vi "Image Caption.vi"(0 "PDF Report IN":T21(xcontrol), 9 "Caption IN":string, 11 "error IN":errorcluster) -> (4 "PDF Report OUT":T21(xcontrol), 6 "Paragraph Refnum":refnum<k24>, 15 "error OUT":errorcluster)   [LabVIEW 2013]
doc: "Version 1.0\nDeveloped by Jean-Marc Simard\nCopyright © 2010, Exaprom Inc.\nAll rights reserved.\nLicense: BSD\n\nWith iTextSharp 4.1.6 (http://itextsharp.sourceforge.net)\nunder Mozilla Public License Version 1.1\n(http://www.mozilla.org/MPL/MPL-1.1.html)"
uses:
  Controls/PDF Report Xcontrol/PDF Report.xctl
  C:/Users/MaxCorp/Documents/GitHub/TopView/DLL/itextsharp.dll
  DLL/itextsharp.dll
  Controls/Paragraphe cluster.ctl
  Controls/Texte alignement.ctl
  Controls/Line spacing.ctl
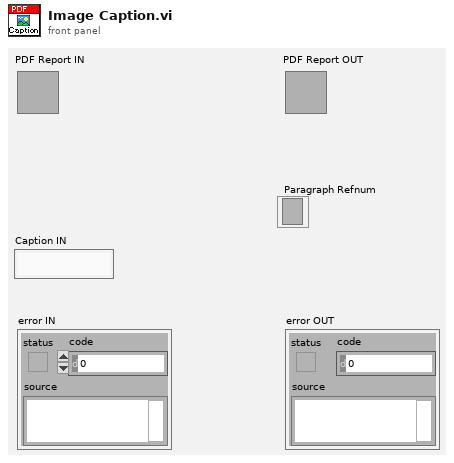
[diagram p1: front panel]
types:
  T1 = typedef "Font cluster.ctl" = cluster{"Name":string, "Size":T2, "Color":T3, "Style":cluster{"Bold":bool, "Italic":bool, "Underline":bool, "Strikeout":bool}}
  T2 = typedef "Font size.ctl" = sgl
  T3 = typedef "Font color.ctl" = u32
  T4 = typedef "Unit.ctl" = enum16{"inch", "mm"}
  T5 = typedef "Paragraphe cluster.ctl" = cluster{" Aligment":T6, "Line spacing":T7}
  T6 = typedef "Texte alignement.ctl" = enum16{"Select", "CENTER", "JUSTIFY", "LEFT", "RIGHT"}
  T7 = typedef "Line spacing.ctl" = enum16{"Select", "1.0", "1.5", "2.0"}
  T8 = typedef "Page dimensions.ctl" = cluster{"Start at page":i32, "Orientation":T9, "widht":sgl, "height":sgl, "Margin left":sgl, "Margin right":sgl, "Margin top":sgl, "Margin bottom":sgl}
  T9 = typedef "Page Orientation.ctl" = enum16{"Portrait", "Landscape"}
  T10 = typedef "Image or Table Caption.ctl" = cluster{"Caption":string, "Separator":string, "Position":enum16{"Above", "Below"}}
  T11 = typedef "Header Footer [ ].ctl" = T12[]
  T12 = typedef "Header Footer cluster.ctl" = cluster{"Start page":i32, "Type":T13, "Alignment":T14, "Vertical Alignement":T15, "Image (%)":sgl, "Page #":T16, "Text":string, "Path":string, "Font":T1, "Font refnum":refnum<k24>, "Line":cluster{"Line":T17, "Thickness (points)":sgl, "Colour":T3}}
  T13 = typedef "Header Footer Type.ctl" = enum16{"Select", "Text", "Text + hyperlink", "Page number", "Image", "Image + hyperlink"}
  T14 = typedef "Header footer horiz alignment.ctl" = enum16{"Left", "Center", "Right"}
  T15 = typedef "Cell Vertical alignment.ctl" = enum16{"TOP", "MIDDLE", "BOTTOM"}
  T16 = typedef "Page number.ctl" = cluster{"Text 1":string, "Text 2":string, "Text 3":string}
  T17 = typedef "Header Footer Line.ctl" = enum16{"No line", "Horizontal line"}
  T18 = typedef "Watermark cluster2.ctl" = cluster{"Show? (F)":bool, "Type":enum16{"Image", "Text"}, "Opacity (%)":sgl, "Rotate(°)":sgl, "Position":cluster{"Position":T19, "X":sgl, "Y":sgl}, "Image path":path, "Scaled(%)":sgl, "Image refnum":refnum<k24>, "Text":string, "Font":cluster{"Name":string, "Size":T2, "Color":T3}, "Font refnum":refnum<k24>, "Alignment":T14, "Automatic":bool}
  T19 = typedef "Watermark Position.ctl" = enum16{"Absolute", "Center (page)", "Center (text section)"}
  T20 = typedef "System Fonts.ctl" = cluster{"Font name [ ]":string[], "Font and file names [ ]":cluster{"Font name":string, "File name":string}[]}
  T21 = cluster{"Document":refnum<k24>, "Writer":refnum<k24>, "Default Font":refnum<k24>, "Default Font cluster":T1, "Path":path, "Unit (default = mm)":T4, "Paragraphe cluster":T5, "Pages dimensions [ ]":T8[], "Captions":cluster{"Image":T10, "Image counter":u16, "Table":T10, "Table counter":u16, "Font":T1}, "Header":T11, "Footer":T11, "Watermark ":T18, "Actual VI name":string, "System Fonts":T20}
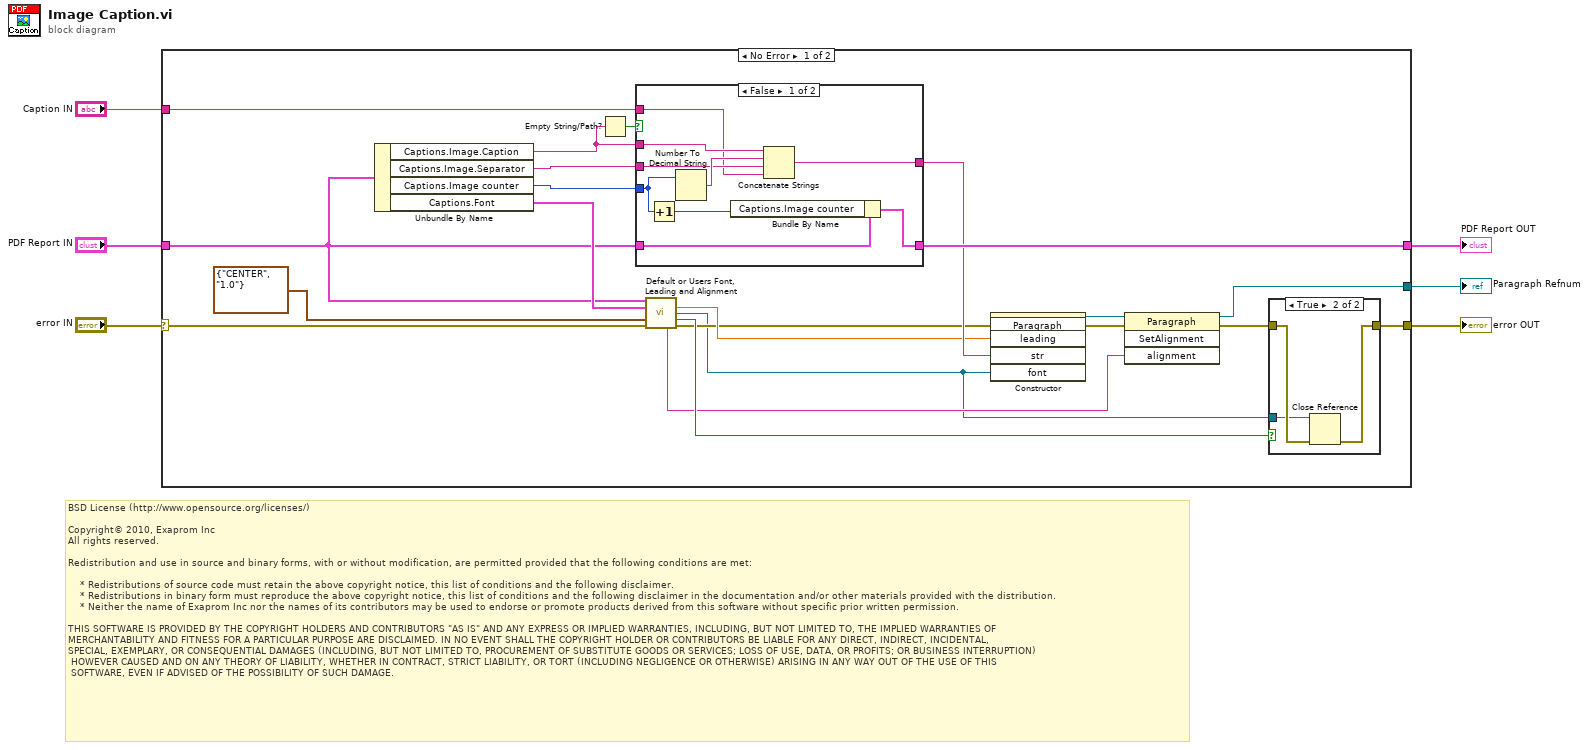
[diagram p0: block diagram]
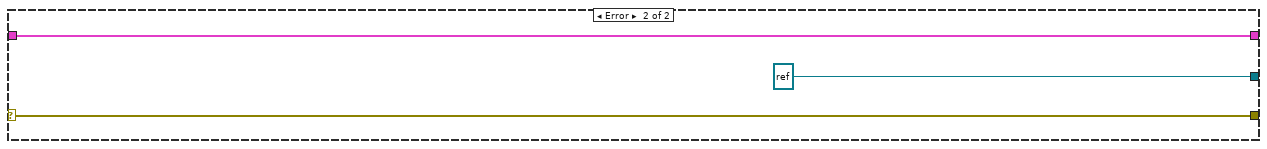
[diagram p4: hidden frame]
diagram:
  # "BSD License (http://www.opensource.org/licenses/)\n\nCopyright© 2010, Exaprom Inc\nAll rights reserved.\n\nRedistribution and use in source and binary forms, with or without modification, are permitted provided that the following conditions are met:\n\n    * Redistributions of source code must retain the above copyright notice, this list of conditions and the following disclaimer.\n    * Redistributions in binary form must reproduce the above copyright notice, this list of conditions and the following disclaimer in the documentation and/or other materials provided with the distribution.\n    * Neither the name of Exaprom Inc nor the names of its contributors may be used to endorse or promote products derived from this software without specific prior written permission.\n\nTHIS SOFTWARE IS PROVIDED BY THE COPYRIGHT HOLDERS AND CONTRIBUTORS \"AS IS\" AND ANY EXPRESS OR IMPLIED WARRANTIES, INCLUDING, BUT NOT LIMITED TO, THE IMPLIED WARRANTIES OF \nMERCHANTABILITY AND FITNESS FOR A PARTICULAR PURPOSE ARE DISCLAIMED. IN NO EVENT SHALL THE COPYRIGHT HOLDER OR CONTRIBUTORS BE LIABLE FOR ANY DIRECT, INDIRECT, INCIDENTAL,\nSPECIAL, EXEMPLARY, OR CONSEQUENTIAL DAMAGES (INCLUDING, BUT NOT LIMITED TO, PROCUREMENT OF SUBSTITUTE GOODS OR SERVICES; LOSS OF USE, DATA, OR PROFITS; OR BUSINESS INTERRUPTION)\n HOWEVER CAUSED AND ON ANY THEORY OF LIABILITY, WHETHER IN CONTRACT, STRICT LIABILITY, OR TORT (INCLUDING NEGLIGENCE OR OTHERWISE) ARISING IN ANY WAY OUT OF THE USE OF THIS\n SOFTWARE, EVEN IF ADVISED OF THE POSSIBILITY OF SUCH DAMAGE."
  n1 = case shown="No Error" "error IN" {
    selector: "error IN" -> [w17 w45]
    tunnel: [w26 w44] -> w6
    tunnel: "Caption IN" -> [w22 _]
    tunnel: "PDF Report IN" -> [w16 w44]
    tunnel: [w19 w45] -> w3
    tunnel: [w7 refnum<k24> refnum ("new reference")] -> w1
    frame No Error {
      n2 = Unbundle By Name(w16) -> ("Captions.Image.Caption"=w23:string, "Captions.Image.Separator"=w24:string, "Captions.Image counter"=w25:u16, "Captions.Font"=w27:T1)
      n3 = Empty String/Path?(string/path=w23) -> (empty?=w21:bool)
      n4 = case shown="False" w21 {
        tunnel: w22 -> [w37 w42]
        tunnel: w23 -> [w40 _]
        tunnel: w24 -> [w38 _]
        tunnel: w25 -> [w36 _]
        tunnel: [w32 w42] -> w13
        tunnel: w16 -> [w35 w41]
        tunnel: [w33 w41] -> w26
        frame False {
          n5 = Increment(x=w36) -> (x+1=w34:u16)
          n6 = Number To Decimal String(number=w36) -> (decimal integer string=w39:string)  [unwired: 1 out]
          n7 = Bundle By Name(cluster=w35, "Captions.Image counter"=w34) -> (w33:T21)
          n8 = Concatenate Strings(w40, w39, w38, w37) -> (w32:string)
        }
        frame True {
        }
      }
      n9 = call "Default or Users Font, Leading and Alignment.vi"("PDF Report"=w16, "Font"=w27, "Paragraphe cluster"=T5 {" Aligment"=enum."CENTER", "Line spacing"=enum."1.0"}, "error in (no error)"=w17) -> ("Leading"=w12:T2, "Font Ref"=w8:refnum<k24>, "Close Font Ref"=w18:bool, "Aligment"=w10:string, "error out"=w11:errorcluster)  [unwired: 7 out]
      n10 = constructor class="Paragraph"(error in=w11, "leading"=w12, "str"=w13, "font"=w8) -> (reference out=w14:refnum<k24>, error out=w15:errorcluster)  [unwired: 2 in, 4 out]
      n11 = invoke class="Paragraph" method="SetAlignment"(reference=w14, error in=w15, "alignment"=w10) -> (reference out=w7:refnum<k24>, error out=w9:errorcluster)  [unwired: 1 in, 2 out]
      n12 = case shown="True" w18 {
        tunnel: w9 -> [w28 w31]
        tunnel: w8 -> [_ w30]
        tunnel: [w28 w29] -> w19
        frame False {
        }
        frame True {
          n13 = Close Reference(reference=w30, error in (no error)=w31) -> (error out=w29:errorcluster)
        }
      }
    }
    frame Error {
    }
  }
  "PDF Report OUT" <- w6
  "error OUT" <- w3
  "Paragraph Refnum" <- w1
